vi "SelectFunction.vi"(10 "Found?":bool, 11 "Library":T1) -> (2 "Version":string, 3 "Function":string)   [LabVIEW 2019, in "ByteLVDevEnv.lvlib"]
doc: "Sets the library function: Install from VIMP, Search in Local Folder, Skip (Already installed)"
uses:
  ByteLVDevEnv.lvlib
  TypeDefs/AllLibraries.ctl
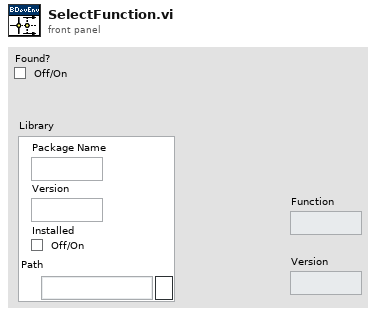
[diagram p1: front panel]
types:
  T1 = typedef "ByteLVDevEnv.lvlib/AllLibraries.ctl" = cluster{"Package Name":string, "Version":string, "Installed":bool, "Path":path}
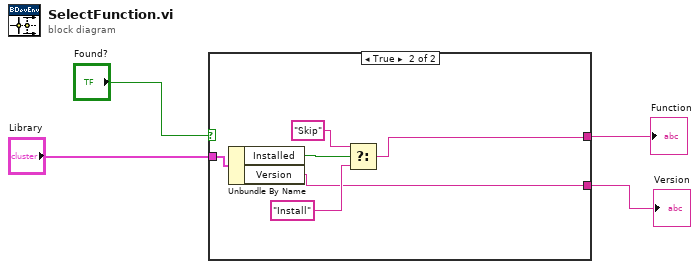
[diagram p0: block diagram]
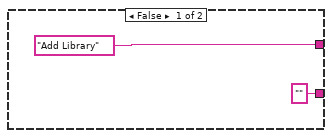
[diagram p2: hidden frame]
diagram:
  n1 = case shown="True" "Found?" {
    tunnel: ["Add Library" w8] -> w3
    tunnel: "Library" -> [_ w12]
    tunnel: ["" ("Version") w7] -> w1
    frame False {
    }
    frame True {
      n2 = Unbundle By Name(w12) -> ("Installed"=w11:bool, "Version"=w7:string)
      n3 = Select(t="Skip", s=w11, f="Install") -> (s? t:f=w8:string)
    }
  }
  "Function" <- w3
  "Version" <- w1
